vi "Test Write.vi"(8 "error in (no error)":errorcluster, 9 "data table":T1, 10 "data dictionary":refnum<class "data dictionary.lvclass">, 11 "runtime in":refnum<class "SystemLink runtime.lvclass">) -> (0 "error out":errorcluster, 1 "Test Number":dbl, 2 "Pass":bool[](array[boolean]), 3 "runtime out":refnum<class "SystemLink runtime.lvclass">)   [LabVIEW 2015, in "SystemLink Tag Module tests.lvlib"]
uses:
  SystemLink Tag Module tests.lvlib
  module/execution/SystemLink runtime.lvclass
  <vilib>/NI/Tag Bus/table/data table.ctl
  <vilib>/NI/Tag Bus/dictionary/data dictionary.lvclass
  <vilib>/Skyline/Tag/Shared/typedefs/DataType.ctl
  <vilib>/NI/Tag Bus/dictionary/data dictionary.lvclass/data dictionary.ctl
  <vilib>/NI/Tag Bus/dictionary/lookup polymorphs/locate double.vi
  <vilib>/NI/Tag Bus/table/data polymorphs/write one/write Double.vi
  <vilib>/NI/Tag Bus/dictionary/lookup polymorphs/locate Single.vi
  <vilib>/NI/Tag Bus/table/data polymorphs/write one/write Single.vi
  <vilib>/NI/Tag Bus/dictionary/lookup polymorphs/locate I32.vi
  <vilib>/NI/Tag Bus/table/data polymorphs/write one/write I32.vi
  <vilib>/NI/Tag Bus/dictionary/lookup polymorphs/locate I16.vi
  <vilib>/NI/Tag Bus/table/data polymorphs/write one/write I16.vi
  <vilib>/NI/Tag Bus/dictionary/lookup polymorphs/locate I8.vi
  <vilib>/NI/Tag Bus/table/data polymorphs/write one/write I8.vi
  <vilib>/NI/Tag Bus/dictionary/lookup polymorphs/locate Boolean.vi
  <vilib>/NI/Tag Bus/table/data polymorphs/write one/write Boolean.vi
  <vilib>/NI/Tag Bus/dictionary/lookup polymorphs/locate String.vi
  <vilib>/NI/Tag Bus/table/data polymorphs/write one/write String.vi
  <vilib>/NI/Tag Bus/dictionary/lookup polymorphs/locate U64.vi
  <vilib>/NI/Tag Bus/table/data polymorphs/write one/write U64.vi
  <vilib>/NI/Tag Bus/dictionary/search/find data index.vi
  <vilib>/NI/Tag Bus/dictionary/search/search string list.vi
  <vilib>/NI/Tag Bus/dictionary/tag not found.vi
  <vilib>/Skyline/Tag/Wrapper/Wrapper AMQP_class/Open Tag AMQP.vi
  <vilib>/Skyline/Tag/Wrapper/Wrapper_class/Read Tag (I32).vi
  <vilib>/Skyline/Tag/Wrapper/Wrapper_class/Close Tag (Single).vi
  <vilib>/Skyline/Tag/Wrapper/Wrapper_class/Read Tag (U64).vi
  <vilib>/Skyline/Tag/Wrapper/Wrapper_class/Read Tag (Boolean).vi
  <vilib>/Skyline/Tag/Wrapper/Wrapper_class/Read Tag (String).vi
  <vilib>/Skyline/Tag/Wrapper/Wrapper_class/Read Tag (DBL).vi
  <vilib>/NI/Tag Bus/table/data table.lvlib
  <vilib>/Skyline/Tag/Wrapper/Wrapper_class/NI Skyline Tag.lvclass
  <vilib>/Skyline/Tag/Wrapper/Wrapper AMQP_class/NI Skyline Tag AMQP.lvclass
  <vilib>/Skyline/Tag/Shared/NI Skyline Tag.lvlib
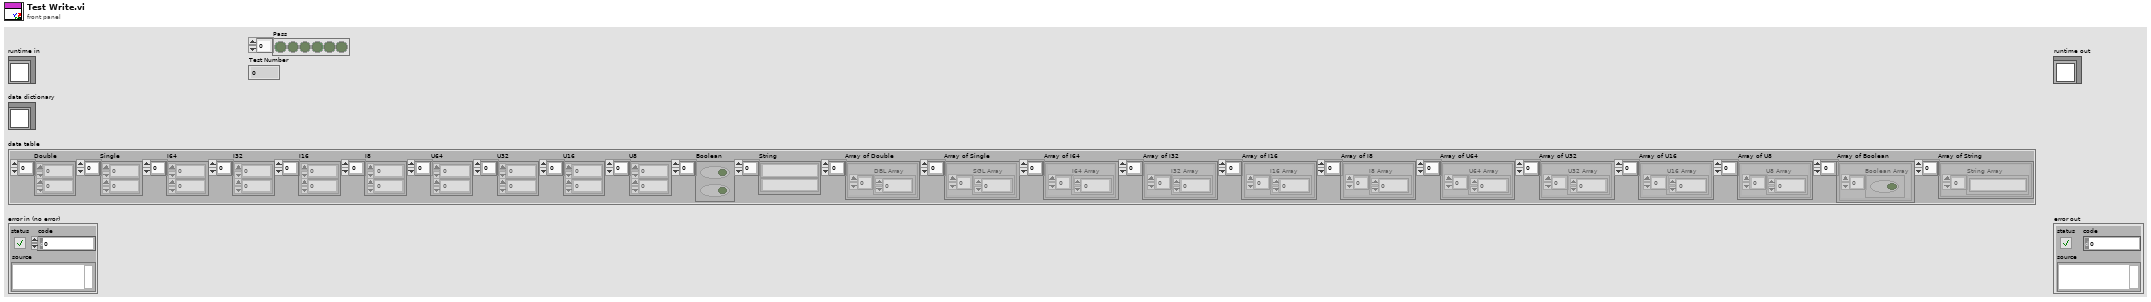
[diagram p1: front panel]
types:
  T1 = typedef "tag bus.lvlib/data table.lvlib/data table.ctl" = cluster{"Double":dbl[], "Single":sgl[], "I64":i64[], "I32":i32[], "I16":i16[], "I8":i8[], "U64":u64[], "U32":u32[], "U16":u16[], "U8":u8[], "Boolean":bool[], "String":string[], "Array of Double":cluster{"DBL Array":dbl[]}[], "Array of Single":cluster{"SGL Array":sgl[]}[], "Array of I64":cluster{"I64 Array":i64[]}[], "Array of I32":cluster{"I32 Array":i32[]}[], "Array of I16":cluster{"I16 Array":i16[]}[], "Array of I8":cluster{"I8 Array":i8[]}[], "Array of U64":cluster{"U64 Array":u64[]}[], "Array of U32":cluster{"U32 Array":u32[]}[], "Array of U16":cluster{"U16 Array":u16[]}[], "Array of U8":cluster{"U8 Array":u8[]}[], "Array of Boolean":cluster{"Boolean Array":bool[]}[], "Array of String":cluster{"String Array":string[]}[]}
  T2 = typedef "NI Skyline Tag.lvlib/DataType.ctl" = enum32{"Double", "I32", "String", "Boolean", "U64", "Timestamp"}
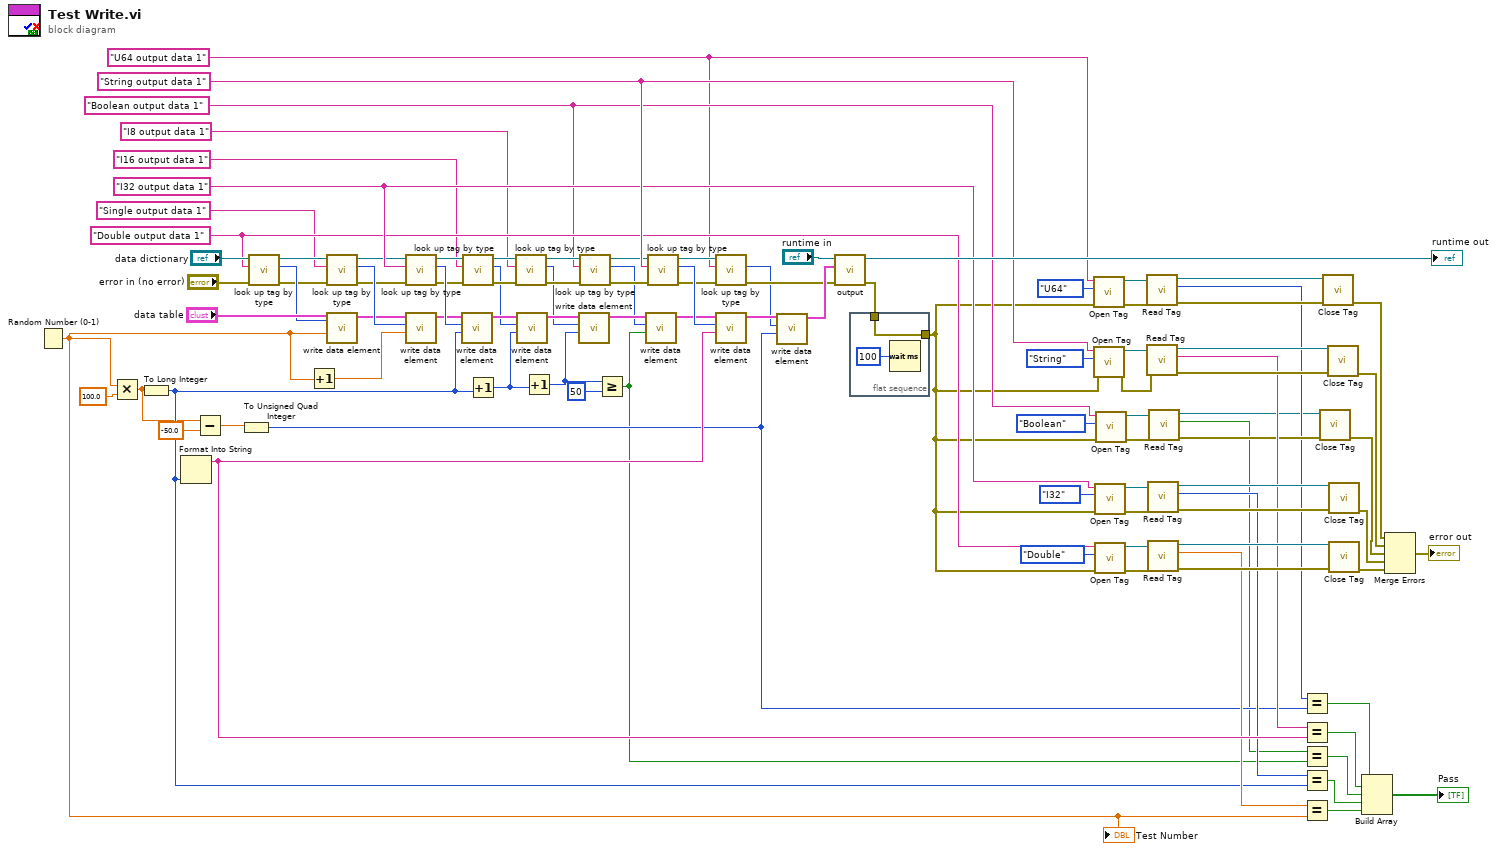
[diagram p0: block diagram]
diagram:
  w6 = "U64 output data 1" ("channel name")
  w28 = "Boolean output data 1" ("channel name")
  w80 = "String output data 1" ("channel name")
  w79 = "I32 output data 1" ("channel name")
  w78 = "Double output data 1" ("channel name")
  n1 = Random Number (0-1)() -> (number: 0 to 1=w39:dbl)
  "Test Number" <- w39
  n2 = Multiply(x=w39, y=100.0) -> (x*y=w19:dbl)
  n3 = To Long Integer(number=w19) -> (32bit integer=w37:i32)
  n4 = Format Into String(w37) -> (resulting string=w76:string)  [unwired: 3 in, 1 out]
  n5 = Subtract(x=w19, y=-50.0) -> (x-y=w17:dbl)
  n6 = To Unsigned Quad Integer(1:w17) -> (0:w11:u64)
  n7 = call-poly <vilib>:"look up tag by type.vi"("error in"="error in (no error)", "name"=w78, "data dictionary in"="data dictionary") -> ("error out"=w63:errorcluster, "index"=w95:i32, "data dictionary out"=w61:refnum<class "data dictionary.lvclass">)  [unwired: 6 in]
  n8 = Increment(x=w39) -> (x+1=w38:dbl)
  n9 = call-poly <vilib>:"look up tag by type.vi"("error in"=w63, "name"="Single output data 1", "data dictionary in"=w61) -> ("error out"=w62:errorcluster, "index"=w64:i32, "data dictionary out"=w60:refnum<class "data dictionary.lvclass">)  [unwired: 6 in]
  n10 = call-poly <vilib>:"write data element.vi"("value"=w39, "index"=w95, "data table in"="data table") -> ("data table out"=w59:T1)  [unwired: 8 in]
  n11 = call-poly <vilib>:"look up tag by type.vi"("error in"=w62, "name"=w79, "data dictionary in"=w60) -> ("error out"=w57:errorcluster, "index"=w100:i32, "data dictionary out"=w56:refnum<class "data dictionary.lvclass">)  [unwired: 6 in]
  n12 = call-poly <vilib>:"write data element.vi"("value"=w38, "index"=w64, "data table in"=w59) -> ("data table out"=w45:T1)  [unwired: 8 in]
  n13 = call-poly <vilib>:"write data element.vi"("value"=w37, "index"=w100, "data table in"=w45) -> ("data table out"=w44:T1)  [unwired: 8 in]
  n14 = call-poly <vilib>:"look up tag by type.vi"("error in"=w57, "name"="I16 output data 1" ("channel name"), "data dictionary in"=w56) -> ("error out"=w55:errorcluster, "index"=w42:i32, "data dictionary out"=w54:refnum<class "data dictionary.lvclass">)  [unwired: 6 in]
  n15 = Increment(x=w37) -> (x+1=w36:i32)
  n16 = call-poly <vilib>:"look up tag by type.vi"("error in"=w55, "name"="I8 output data 1" ("channel name"), "data dictionary in"=w54) -> ("error out"=w53:errorcluster, "index"=w41:i32, "data dictionary out"=w52:refnum<class "data dictionary.lvclass">)  [unwired: 6 in]
  n17 = call-poly <vilib>:"write data element.vi"("value"=w36, "index"=w42, "data table in"=w44) -> ("data table out"=w47:T1)  [unwired: 8 in]
  n18 = Increment(x=w36) -> (x+1=w35:i32)
  n19 = call-poly <vilib>:"write data element.vi"("value"=w35, "index"=w41, "data table in"=w47) -> ("data table out"=w46:T1)  [unwired: 8 in]
  n20 = call-poly <vilib>:"look up tag by type.vi"("error in"=w53, "name"=w28, "data dictionary in"=w52) -> ("error out"=w50:errorcluster, "index"=w40:i32, "data dictionary out"=w51:refnum<class "data dictionary.lvclass">)  [unwired: 6 in]
  n21 = Greater Or Equal?(x=w35, y=50) -> (x >= y?=w7:bool)
  n22 = call-poly <vilib>:"write data element.vi"("value"=w7, "index"=w40, "data table in"=w46) -> ("data table out"=w43:T1)  [unwired: 8 in]
  n23 = call-poly <vilib>:"look up tag by type.vi"("error in"=w50, "name"=w80, "data dictionary in"=w51) -> ("error out"=w23:errorcluster, "index"=w101:i32, "data dictionary out"=w21:refnum<class "data dictionary.lvclass">)  [unwired: 6 in]
  n24 = call-poly <vilib>:"look up tag by type.vi"("error in"=w23, "name"=w6, "data dictionary in"=w21) -> ("error out"=w22:errorcluster, "index"=w20:i32)  [unwired: 6 in, 1 out]
  n25 = call-poly <vilib>:"write data element.vi"("value"=w76, "index"=w101, "data table in"=w43) -> ("data table out"=w25:T1)  [unwired: 8 in]
  n26 = call-poly <vilib>:"write data element.vi"("value"=w11, "index"=w20, "data table in"=w25) -> ("data table out"=w24:T1)  [unwired: 8 in]
  n27 = call-dynamic "output.vi"("error in"=w22, "data table in"=w24, "SystemLin Tag Module runtime in"="runtime in") -> ("error out"=w3:errorcluster, "SystemLin Tag Module runtime out"=→"runtime out":refnum<class "SystemLink runtime.lvclass">)  [unwired: 6 in, 1 out]
  n28 = flat-sequence {
    tunnel: [w102] -> w2
    tunnel: w3 -> [w102]
    frame #0 {
      n29 = Wait (ms)(milliseconds to wait=u32 100) -> ()  [unwired: 1 out]
    }
  }
  n30 = call-poly <vilib>:"Open Tag.vi"("error in (no error)"=w2, "data type"=DataType."U64", "path"=w6) -> ("error out"=w30:errorcluster, "tag out"=w13:refnum<class "NI Skyline Tag.lvclass">)  [unwired: 7 in]
  n31 = call-poly <vilib>:"Open Tag.vi"("error in (no error)"=w2, "data type"=DataType."String", "path"=w80) -> ("error out"=w91:errorcluster, "tag out"=w92:refnum<class "NI Skyline Tag.lvclass">)  [unwired: 7 in]
  n32 = call-poly <vilib>:"Open Tag.vi"("error in (no error)"=w2, "data type"=DataType."I32", "path"=w79) -> ("error out"=w86:errorcluster, "tag out"=w85:refnum<class "NI Skyline Tag.lvclass">)  [unwired: 7 in]
  n33 = call-poly <vilib>:"Open Tag.vi"("error in (no error)"=w2, "data type"=DataType."Double", "path"=w78) -> ("error out"=w83:errorcluster, "tag out"=w84:refnum<class "NI Skyline Tag.lvclass">)  [unwired: 7 in]
  n34 = call-poly <vilib>:"Open Tag.vi"("error in (no error)"=w2, "data type"=DataType."Boolean", "path"=w28) -> ("error out"=w31:errorcluster, "tag out"=w5:refnum<class "NI Skyline Tag.lvclass">)  [unwired: 7 in]
  n35 = call-poly <vilib>:"Read Tag.vi"("error in (no error)"=w30, "tag in"=w13) -> ("error out"=w15:errorcluster, "value"=w12:u64, "tag out"=w14:refnum<class "NI Skyline Tag.lvclass">)  [unwired: 5 in, 2 out]
  n36 = call-poly <vilib>:"Read Tag.vi"("error in (no error)"=w91, "tag in"=w92) -> ("error out"=w90:errorcluster, "value"=w77:string, "tag out"=w89:refnum<class "NI Skyline Tag.lvclass">)  [unwired: 5 in, 2 out]
  n37 = call-poly <vilib>:"Read Tag.vi"("error in (no error)"=w86, "tag in"=w85) -> ("error out"=w87:errorcluster, "value"=w75:i32, "tag out"=w88:refnum<class "NI Skyline Tag.lvclass">)  [unwired: 5 in, 2 out]
  n38 = call-poly <vilib>:"Read Tag.vi"("error in (no error)"=w83, "tag in"=w84) -> ("error out"=w82:errorcluster, "value"=w74:dbl, "tag out"=w81:refnum<class "NI Skyline Tag.lvclass">)  [unwired: 5 in, 2 out]
  n39 = call-poly <vilib>:"Read Tag.vi"("error in (no error)"=w31, "tag in"=w5) -> ("error out"=w27:errorcluster, "value"=w8:bool, "tag out"=w4:refnum<class "NI Skyline Tag.lvclass">)  [unwired: 5 in, 2 out]
  n40 = Equal?(x=w12, y=w11) -> (x = y?=w10:bool)
  n41 = Equal?(x=w77, y=w76) -> (x = y?=w73:bool)
  n42 = Equal?(x=w8, y=w7) -> (x = y?=w9:bool)
  n43 = Equal?(x=w75, y=w37) -> (x = y?=w72:bool)
  n44 = Equal?(x=w74, y=w39) -> (x = y?=w71:bool)
  n45 = call-poly <vilib>:"Close Tag.vi"("error in (no error)"=w27, "tag in"=w4) -> ("error out"=w26:errorcluster)  [unwired: 9 in]
  n46 = call-poly <vilib>:"Close Tag.vi"("error in (no error)"=w15, "tag in"=w14) -> ("error out"=w16:errorcluster)  [unwired: 9 in]
  n47 = call-poly <vilib>:"Close Tag.vi"("error in (no error)"=w90, "tag in"=w89) -> ("error out"=w67:errorcluster)  [unwired: 9 in]
  n48 = call-poly <vilib>:"Close Tag.vi"("error in (no error)"=w87, "tag in"=w88) -> ("error out"=w66:errorcluster)  [unwired: 9 in]
  n49 = call-poly <vilib>:"Close Tag.vi"("error in (no error)"=w82, "tag in"=w81) -> ("error out"=w65:errorcluster)  [unwired: 9 in]
  n50 = Build Array(w10, w73, w9, w72, w71) -> (→"Pass":bool[])
  n51 = Merge Errors(w16, w67, w26, w66, w65) -> (→"error out":errorcluster)
